vi "set value BOOL.vi"(8 "error in (no error)":errorcluster, 10 "Payload":cluster{"name":string, "value":bool}, 11 "VI Ref":refnum<vi>) -> (0 "error out":errorcluster, 3 "return value":string)   [LabVIEW 2020, in "ui-testing.lvlib"]
uses:
  ui-testing.lvlib
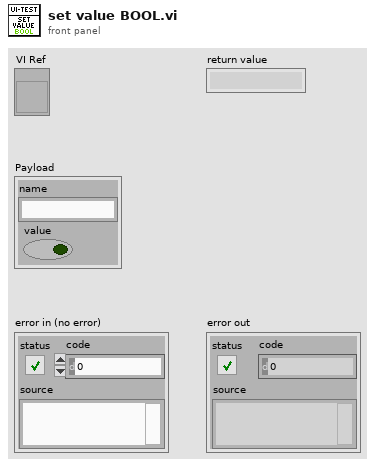
[diagram p1: front panel]
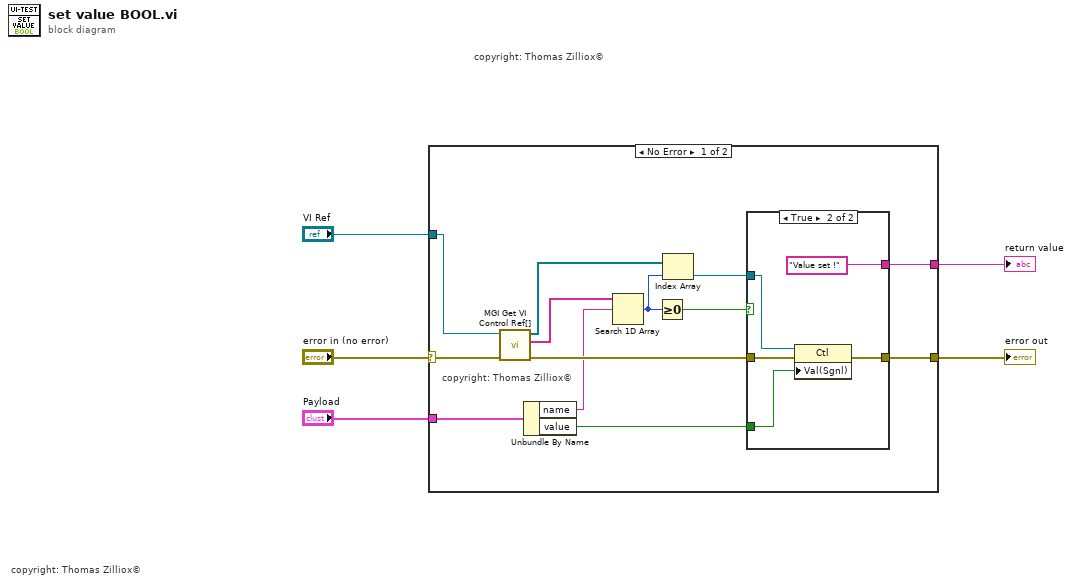
[diagram p0: block diagram]
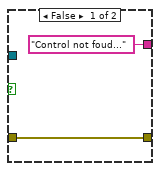
[diagram p2: hidden frame]
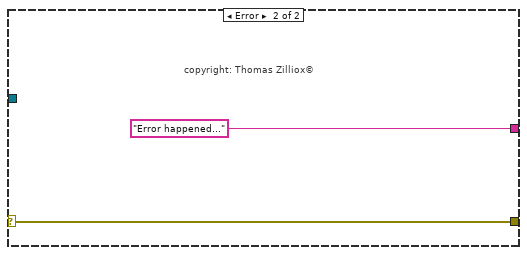
[diagram p3: hidden frame]
diagram:
  # "copyright: Thomas Zilliox©"
  # "copyright: Thomas Zilliox©"
  n1 = case shown="No Error" "error in (no error)" {
    selector: "error in (no error)" -> [w10 w27]
    tunnel: [w16 w27] -> w4
    tunnel: [w17 "Error happened..."] -> w3
    tunnel: "VI Ref" -> [w11 _]
    tunnel: "Payload" -> [w15 _]
    frame No Error {
      # "copyright: Thomas Zilliox©"
      n2 = call <userlib>:"MGI Get VI Control Ref[].vi"("error in"=w10, "VI (Caller)"=w11) -> ("error out"=w9:errorcluster, "Control Label Chain[i]"=w13:string[], "Control[i]"=w12:refnum<vi>[])  [unwired: 6 in, 1 out]
      n3 = Unbundle By Name(w15) -> ("name"=w8:string, "value"=w18:bool)
      n4 = Search 1D Array(1D array=w13, element=w8) -> (index of element=w14:i32)  [unwired: 1 in]
      n5 = Greater Or Equal To 0?(x=w14) -> (x >= 0?=w7:bool)
      n6 = Index Array(array=w12, index=w14) -> (element=w6:refnum<vi>)
      n7 = case shown="True" w7 {
        tunnel: w9 -> [w20 w25]
        tunnel: w18 -> [_ w24]
        tunnel: [w20 w23] -> w16
        tunnel: ["Control not foud..." "Value set !"] -> w17
        tunnel: w6 -> [_ w21]
        frame False {
        }
        frame True {
          n8 = property class="Ctl"(reference=w21, error in=w25, "Val(Sgnl)"=w24) -> (error out=w23:errorcluster)  [unwired: 1 out]
        }
      }
    }
    frame Error {
      # "copyright: Thomas Zilliox©"
    }
  }
  "error out" <- w4
  "return value" <- w3
